vi "svx_Waterfall QueueToState.vi"(11 "State In":T1={"X Scale Width %"=50.0, "Y Scale Height %"=50.0, "X-Axis Range"={"Minimum"=0.0, "Maximum"=10.0}, "Y-Axis Range"={"Minimum"=0.0, "Maximum"=10.0}, "Z-Axis Range"={"Minimum"=0.0, "Maximum"=10.0}, "Plot Color"=61212, "Frame Color"=16252785, "Background Color"=16777222, "Initial AutoScale Y"=TRUE, "AutoScale X"=2, "AutoScale Y"=2, "AutoScale Z"=2, "Plot Transparency"=FALSE, "X-Axis Name"="Frequency", "Y-Axis Name"="Amplitude", "Z-Axis Name"="", "X-Axis Scaling Factor"={"Offset"=0.0, "Multiplier"=1.0}, "Y-Axis Scaling Factor"={"Offset"=0.0, "Multiplier"=1.0}, "Z-Axis Scaling Factor"={"Offset"=0.0, "Multiplier"=1.0}, "X-Scale Visible"=TRUE, "Y-Scale Visible"=TRUE, "Z-Scale Visible"=TRUE, "X-Scale Label Visible"=TRUE, "Y-Scale Label Visible"=TRUE, "Z-Scale Label Visible"=TRUE, "X-Axis Range Scaled"={"Minimum"=0.0, "Maximum"=10.0}, "Y-Axis Range Scaled"={"Minimum"=0.0, "Maximum"=10.0}, "Z-Axis Range Scaled"={"Minimum"=0.0, "Maximum"=10.0}, "Rev Z Order"=FALSE, "X-Scale Format Str"="%#.4g", "Y-Scale Format Str"="%#.4g", "Z-Scale Format Str"="%#.4g", "Decor color"=12369084, "Scale Range Change"=refnum, "out of state queue"=refnum, "property nodes"=refnum, "Lines"=[], "Line Properties"={"Line Color"=61212, "Line Width"=61212, "Line Style"=enum."Dash", "DisplayLines"=FALSE}} {"Line Properties"."Line Width" min=1}) -> (3 "State Out":T1={"X Scale Width %"=50.0, "Y Scale Height %"=50.0, "X-Axis Range"={"Minimum"=0.0, "Maximum"=10.0}, "Y-Axis Range"={"Minimum"=0.0, "Maximum"=10.0}, "Z-Axis Range"={"Minimum"=0.0, "Maximum"=10.0}, "Plot Color"=61212, "Frame Color"=16252785, "Background Color"=16777222, "Initial AutoScale Y"=TRUE, "AutoScale X"=2, "AutoScale Y"=2, "AutoScale Z"=2, "Plot Transparency"=FALSE, "X-Axis Name"="Frequency", "Y-Axis Name"="Amplitude", "Z-Axis Name"="", "X-Axis Scaling Factor"={"Offset"=0.0, "Multiplier"=1.0}, "Y-Axis Scaling Factor"={"Offset"=0.0, "Multiplier"=1.0}, "Z-Axis Scaling Factor"={"Offset"=0.0, "Multiplier"=1.0}, "X-Scale Visible"=TRUE, "Y-Scale Visible"=TRUE, "Z-Scale Visible"=TRUE, "X-Scale Label Visible"=TRUE, "Y-Scale Label Visible"=TRUE, "Z-Scale Label Visible"=TRUE, "X-Axis Range Scaled"={"Minimum"=0.0, "Maximum"=10.0}, "Y-Axis Range Scaled"={"Minimum"=0.0, "Maximum"=10.0}, "Z-Axis Range Scaled"={"Minimum"=0.0, "Maximum"=10.0}, "Rev Z Order"=FALSE, "X-Scale Format Str"="%#.4g", "Y-Scale Format Str"="%#.4g", "Z-Scale Format Str"="%#.4g", "Decor color"=12369084, "Scale Range Change"=refnum, "out of state queue"=refnum, "property nodes"=refnum, "Lines"=[], "Line Properties"={"Line Color"=61212, "Line Width"=61212, "Line Style"=enum."Dash", "DisplayLines"=FALSE}} {"Line Properties"."Line Width" min=1})   [LabVIEW 2017, in "SVX Waterfall Graph.xctl"]
uses:
  <vilib>/addons/_XControls/Waterfall Graph/SVX Waterfall Graph.xctl
  <vilib>/addons/_XControls/Waterfall Graph/subVIs/svx_Waterfall State.ctl
  <vilib>/addons/_NISVFA/_Shared subVIs/Controls/svc_Cluster of Array of Cluster of XYZ.ctl
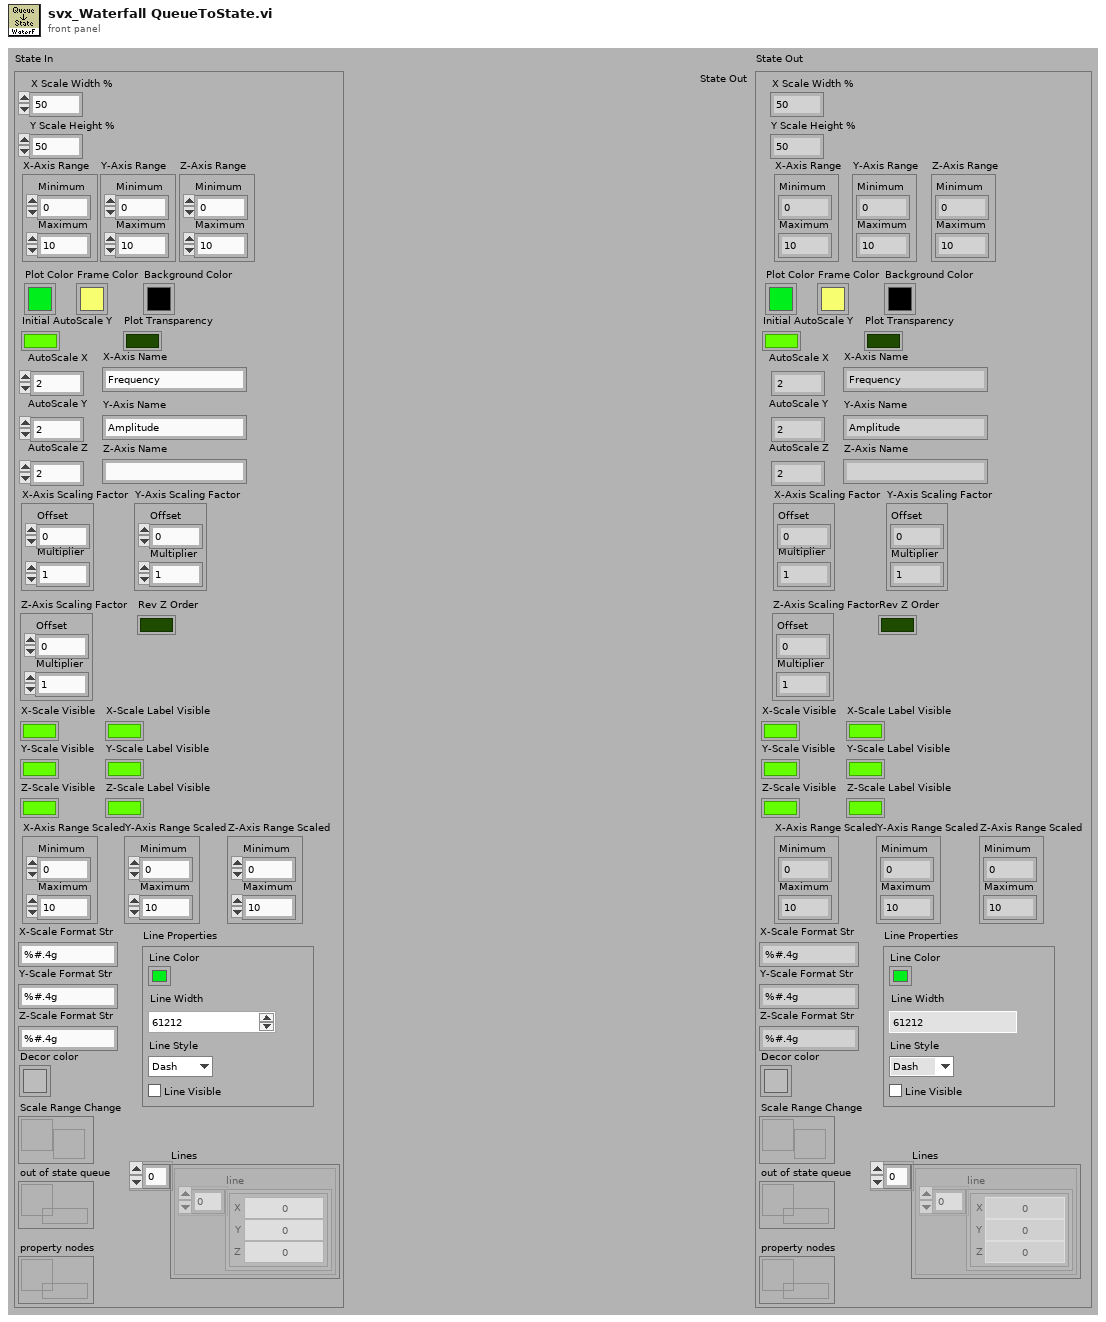
[diagram p1: front panel]
types:
  T1 = typedef "SVX Waterfall Graph.xctl/svx_Waterfall State.ctl" = cluster{"X Scale Width %":dbl, "Y Scale Height %":dbl, "X-Axis Range":cluster{"Minimum":dbl, "Maximum":dbl}, "Y-Axis Range":cluster{"Minimum":dbl, "Maximum":dbl}, "Z-Axis Range":cluster{"Minimum":dbl, "Maximum":dbl}, "Plot Color":u32, "Frame Color":u32, "Background Color":u32, "Initial AutoScale Y":bool, "AutoScale X":u8, "AutoScale Y":u8, "AutoScale Z":u8, "Plot Transparency":bool, "X-Axis Name":string, "Y-Axis Name":string, "Z-Axis Name":string, "X-Axis Scaling Factor":cluster{"Offset":dbl, "Multiplier":dbl}, "Y-Axis Scaling Factor":cluster{"Offset":dbl, "Multiplier":dbl}, "Z-Axis Scaling Factor":cluster{"Offset":dbl, "Multiplier":dbl}, "X-Scale Visible":bool, "Y-Scale Visible":bool, "Z-Scale Visible":bool, "X-Scale Label Visible":bool, "Y-Scale Label Visible":bool, "Z-Scale Label Visible":bool, "X-Axis Range Scaled":cluster{"Minimum":dbl, "Maximum":dbl}, "Y-Axis Range Scaled":cluster{"Minimum":dbl, "Maximum":dbl}, "Z-Axis Range Scaled":cluster{"Minimum":dbl, "Maximum":dbl}, "Rev Z Order":bool, "X-Scale Format Str":string, "Y-Scale Format Str":string, "Z-Scale Format Str":string, "Decor color":u32, "Scale Range Change":refnum<user-event>, "out of state queue":refnum<queue>, "property nodes":refnum<queue>, "Lines":T2[], "Line Properties":cluster{"Line Color":u32, "Line Width":u16, "Line Style":enum32{"Solid", "Dash", "Dot", "DashDot", "DashDotDot"}, "DisplayLines":bool}}
  T2 = typedef "svc_Cluster of Array of Cluster of XYZ.ctl" = cluster{"line":cluster{"X":dbl, "Y":dbl, "Z":dbl}[]}
  T3 = cluster{"use queue?":bool, "X-Axis Range":cluster{"Minimum":dbl, "Maximum":dbl}, "Y-Axis Range":cluster{"Minimum":dbl, "Maximum":dbl}, "Z-Axis Range":cluster{"Minimum":dbl, "Maximum":dbl}, "X-Axis Range Scaled":cluster{"Minimum":dbl, "Maximum":dbl}, "Y-Axis Range Scaled":cluster{"Minimum":dbl, "Maximum":dbl}, "Z-Axis Range Scaled":cluster{"Minimum":dbl, "Maximum":dbl}, "AutoScale X":u8, "AutoScale Y":u8, "AutoScale Z":u8, "background":refnum<vi>}
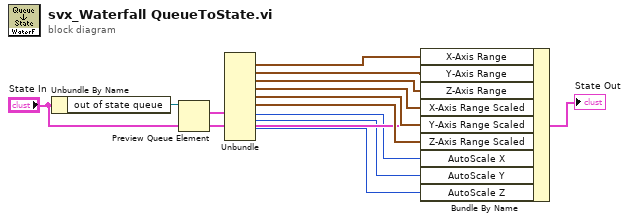
[diagram p0: block diagram]
diagram:
  n1 = Unbundle By Name("State In") -> ("out of state queue"=w9:refnum<queue>)
  n2 = Preview Queue Element(queue=w9) -> (element=w4:T3)  [unwired: 2 in, 3 out]
  n3 = Unbundle(w4) -> ("X-Axis Range"=w7:cluster{"Minimum":dbl, "Maximum":dbl}, "Y-Axis Range"=w8:cluster{"Minimum":dbl, "Maximum":dbl}, "Z-Axis Range"=w13:cluster{"Minimum":dbl, "Maximum":dbl}, "X-Axis Range Scaled"=w12:cluster{"Minimum":dbl, "Maximum":dbl}, "Y-Axis Range Scaled"=w11:cluster{"Minimum":dbl, "Maximum":dbl}, "Z-Axis Range Scaled"=w10:cluster{"Minimum":dbl, "Maximum":dbl}, "AutoScale X"=w3:u8, "AutoScale Y"=w2:u8, "AutoScale Z"=w1:u8)  [unwired: 2 out]
  n4 = Bundle By Name(cluster="State In", "X-Axis Range"=w7, "Y-Axis Range"=w8, "Z-Axis Range"=w13, "X-Axis Range Scaled"=w12, "Y-Axis Range Scaled"=w11, "Z-Axis Range Scaled"=w10, "AutoScale X"=w3, "AutoScale Y"=w2, "AutoScale Z"=w1) -> (→"State Out":T1)
